vi "Read Assertion Results.vi"(11 "Method Result In":refnum<class "Method Result.lvclass">) -> (2 "Assertion Results":refnum<class "Assertion Result.lvclass">[](array[class]), 3 "Method Result Out":refnum<class "Method Result.lvclass">)   [LabVIEW 2020, in "Method Result.lvclass"]
uses:
  Method Result.lvclass
  Assertion Result/Assertion Result.lvclass
  Method Result.lvclass/Method Result.ctl
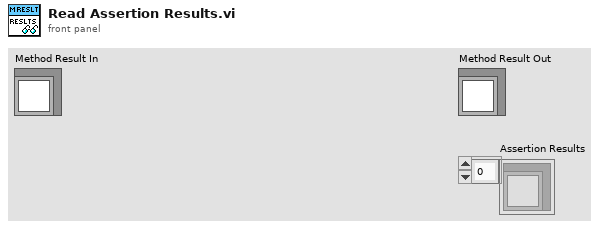
[diagram p1: front panel]
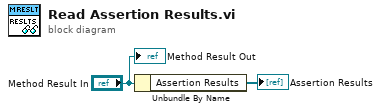
[diagram p0: block diagram]
diagram:
  n1 = Unbundle By Name("Method Result In") -> ("Assertion Results"=→"Assertion Results":refnum<class "Assertion Result.lvclass">[])
  "Method Result Out" <- "Method Result In"
